vi "ISX3_Parse_Channel.vi"(0 "Array":u8[](array[numeric])) -> (1 "Measuremode":u8, 2 "Measurement Channel":u8, 3 "Range Settings":u8)   [LabVIEW 2012, in "Sciospec ISX3 Impedance Analyzer.lvlib"]
uses:
  Sciospec ISX3 Impedance Analyzer.lvlib
panel:
  # "This VI parses a data frame that contains channel settings"
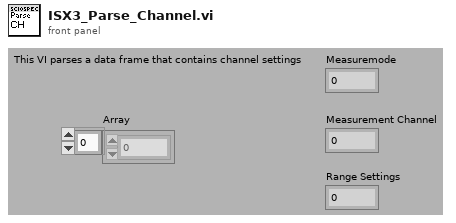
[diagram p1: front panel]
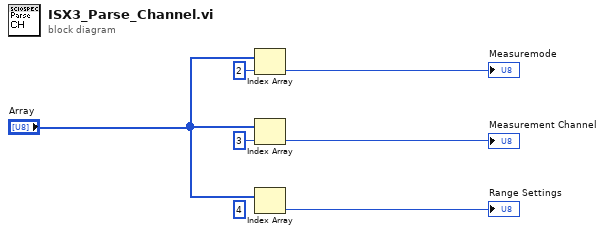
[diagram p0: block diagram]
diagram:
  (unwired) 4 ("Index")
  n1 = Index Array(array="Array", index=2 ("Index")) -> (element=→"Measuremode":u8)
  n2 = Index Array(array="Array", index=3 ("Index")) -> (element=→"Measurement Channel":u8)
  n3 = Index Array(array="Array") -> (element=→"Range Settings":u8)  [unwired: 1 in]
